vi "FOCUS_V42.vi"(9 "X-pixels":sgl=256.0, 11 "Run":bool) -> (0 "Retrace pixels":sgl, 10 "Pixel Clock (Hz)":sgl)   [LabVIEW 2010] (continued)
                  n1367 = property on="index (row)1" class="Slide (strict)"("Scale.Range:Minimum"=w940, "Scale.Range:Maximum"=w941) -> ()  [unwired: 2 in, 2 out]
                  n1368 = Add(x=w956, y=w957) -> (x+y=w955:dbl)
                  n1369 = property on="Histogram2" class="XYGraph (strict)"("X Scale.Range:Minimum"=w956, "X Scale.Range:Maximum"=w955) -> ()  [unwired: 2 in, 2 out]
                  n1370 = property on="Histogram1" class="XYGraph (strict)"("X Scale.Range:Minimum"=w956, "X Scale.Range:Maximum"=w955) -> ()  [unwired: 2 in, 2 out]
                  n1371 = Initialize Array(u32 0 ("element"), w891) -> (w949:u32[])
                  n1372 = Array Subset(array=w887, index (row)=w902, length (row)=w901) -> (w947:u8[][])  [unwired: 2 in]
                  n1373 = Initialize Array(u32 0 ("element"), w891) -> (w953:u32[])
                  n1374 = Array Subset(array=w886, index (row)=w900, length (row)=w899) -> (w951:u8[][])  [unwired: 2 in]
                  n1375 = property on="index (row)2" class="Slide (strict)"("Scale.Range:Minimum"=w940, "Scale.Range:Maximum"=w939) -> ()  [unwired: 2 in, 2 out]
                  n1376 = local read "Background1"() -> (w913:bool)
                  n1377 = for {
                    tunnel: w947 -> [w1024] mode=indexing
                    shift-right: [w1023] -> w948
                    shift-left: w949 -> [w1025]
                    n1378 = Add(x=w1025, y=w1024) -> (x+y=w1023:u32[])
                  }
                  n1379 = local read "Index1"() -> (w927:dbl)
                  n1380 = local read "Length1"() -> (w928:dbl)
                  n1381 = for {
                    tunnel: w951 -> [w1021] mode=indexing
                    shift-right: [w1020] -> w952
                    shift-left: w953 -> [w1022]
                    n1382 = Add(x=w1022, y=w1021) -> (x+y=w1020:u32[])
                  }
                  n1383 = local read "X-pixels"() -> (w889:sgl)
                  n1384 = local read "Pixel Clock (Hz)"() -> (w945:sgl)
                  n1385 = Divide(x=w948, y=w901) -> (x/y=w890:dbl[])
                  n1386 = Array Subset(array=w890, index=w927, length=w928) -> (w924:dbl[])
                  n1387 = Divide(x=w952, y=w899) -> (x/y=w930:dbl[])
                  n1388 = Array Subset(array=w887, index (row)=w956, length (row)=w957, index (col)=w903, length (col)=w888) -> (w959:u8[][])
                  n1389 = Array Subset(array=w886, index (row)=w956, length (row)=w957, index (col)=w903, length (col)=w888) -> (w958:u8[][])
                  n1390 = case shown="True" w913 {
                    tunnel: w890 -> [_ w967]
                    frame False {
                    }
                    frame True {
                      n1391 = Array Size(array=w967) -> (size(s)=w968:i32)
                      n1392 = Add Array Elements(numeric array=w967) -> (sum=w969:dbl)
                      n1393 = Divide(x=w969, y=w968) -> (x/y=w966:dbl)
                      n1394 = local write "Background1 2"(w966) -> ()
                    }
                  }
                  n1395 = Array Size(array=w924) -> (size(s)=w926:i32)
                  n1396 = Add Array Elements(numeric array=w924) -> (sum=w925:dbl)
                  n1397 = Divide(x=w889, y=w945) -> (x/y=w944:sgl)
                  n1398 = local write "Image 1"(w959) -> ()
                  n1399 = Divide(x=w925, y=w926) -> (x/y=w912:dbl)
                  n1400 = local write "Image 2"(w958) -> ()
                  n1401 = local write "F01 2"(w912) -> ()
                  n1402 = Multiply(x=1000.0, y=w944) -> (x*y=w894:dbl)
                  n1403 = Multiply(x=w891, y=w894) -> (x*y=w936:dbl)
                  n1404 = case shown="True" w914 {
                    tunnel: w936 -> [_ w1019]
                    frame False {
                    }
                    frame True {
                      n1405 = property on="Profile1" class="XYGraph (strict)"("X Scale.Range:Minimum"=0.0, "X Scale.Range:Maximum"=w1019, "Y Scale.Range:Minimum"=0.0, "Y Scale.Range:Maximum"=255.0) -> ()  [unwired: 2 in, 2 out]
                    }
                  }
                  n1406 = case shown="True" w915 {
                    tunnel: w936 -> [_ w996]
                    frame False {
                    }
                    frame True {
                      n1407 = property on="Profile2" class="XYGraph (strict)"("X Scale.Range:Minimum"=0.0, "X Scale.Range:Maximum"=w996, "Y Scale.Range:Minimum"=0.0, "Y Scale.Range:Maximum"=255.0) -> ()  [unwired: 2 in, 2 out]
                    }
                  }
                  n1408 = local read "F0 1"() -> (w907:bool)
                  n1409 = Multiply(x=w894, y=w942) -> (x*y=w896:dbl[])
                  n1410 = Multiply(x=w894, y=w942) -> (x*y=w954:dbl[])
                  n1411 = local read "F0 2"() -> (w908:bool)
                  n1412 = local read "Background2"() -> (w910:bool)
                  n1413 = case shown="True" w908 {
                    tunnel: w930 -> [w1000 w1014]
                    tunnel: [w1000 w1006] -> w938
                    tunnel: w904 -> [w999 _]
                    tunnel: [w997 i8 -1 ("Active Cursor")] -> w937
                    frame False {
                      n1414 = Less Than 0?(x=w999) -> (x < 0?=w998:bool)
                      n1415 = case shown="False" w998 {
                        selector: w998 -> [w1002 w1004]
                        tunnel: [i8 1 ("Active Cursor") i8 1 ("Active Cursor")] -> w997
                        frame False {
                          n1416 = local write "Reset2"(w1002) -> ()
                        }
                        frame True {
                          n1417 = local write "Reset2"(w1004) -> ()
                        }
                      }
                    }
                    frame True {
                      n1418 = local read "Background2 2"() -> (w1012:sgl)
                      n1419 = local read "F02 2"() -> (w1009:sgl)
                      n1420 = Subtract(x=w1014, y=w1009) -> (x-y=w1013:dbl[])
                      n1421 = Subtract(x=w1009, y=w1012) -> (x-y=w1015:sgl)
                      n1422 = Divide(x=w1013, y=w1015) -> (x/y=w1007:dbl[])
                      n1423 = property on="Profile2" class="XYGraph (strict)"("Y Scale.Range:Minimum"=-100.0, "Y Scale.Range:Maximum"=100.0) -> ()  [unwired: 2 in, 2 out]
                      n1424 = Multiply(x=w1007, y=100.0 ("Y Scale.Range:Maximum")) -> (x*y=w1006:dbl[])
                    }
                  }
                  n1425 = case shown="True" w907 {
                    tunnel: w890 -> [w973 w987]
                    tunnel: [w973 w979] -> w895
                    tunnel: w905 -> [w972 _]
                    tunnel: [w970 i8 -1 ("Active Cursor")] -> w929
                    frame False {
                      n1426 = Less Than 0?(x=w972) -> (x < 0?=w971:bool)
                      n1427 = case shown="True" w971 {
                        selector: w971 -> [w975 w977]
                        tunnel: [i8 1 ("Active Cursor") i8 1 ("Active Cursor")] -> w970
                        frame False {
                          n1428 = local write "Reset1"(w975) -> ()
                        }
                        frame True {
                          n1429 = local write "Reset1"(w977) -> ()
                        }
                      }
                    }
                    frame True {
                      n1430 = local read "Background1 2"() -> (w985:sgl)
                      n1431 = local read "F01 2"() -> (w982:sgl)
                      n1432 = Subtract(x=w987, y=w982) -> (x-y=w986:dbl[])
                      n1433 = Subtract(x=w982, y=w985) -> (x-y=w988:sgl)
                      n1434 = Divide(x=w986, y=w988) -> (x/y=w980:dbl[])
                      n1435 = property on="Profile1" class="XYGraph (strict)"("Y Scale.Range:Minimum"=-100.0, "Y Scale.Range:Maximum"=100.0) -> ()  [unwired: 2 in, 2 out]
                      n1436 = Multiply(x=w980, y=100.0 ("Y Scale.Range:Maximum")) -> (x*y=w979:dbl[])
                    }
                  }
                  n1437 = property on="Profile2" class="XYGraph (strict)"() -> ("X Scale.Range:Minimum"=w919:dbl, "X Scale.Range:Maximum"=w918:dbl)  [unwired: 2 in, 2 out]
                  n1438 = local read "Index2"() -> (w932:dbl)
                  n1439 = local read "Length2"() -> (w931:dbl)
                  n1440 = property on="Profile1" class="XYGraph (strict)"() -> ("X Scale.Range:Minimum"=w920:dbl, "X Scale.Range:Maximum"=w921:dbl)  [unwired: 2 in, 2 out]
                  n1441 = case shown="True" w910 {
                    tunnel: w930 -> [_ w990]
                    frame False {
                    }
                    frame True {
                      n1442 = Array Size(array=w990) -> (size(s)=w991:i32)
                      n1443 = Add Array Elements(numeric array=w990) -> (sum=w992:dbl)
                      n1444 = Divide(x=w992, y=w991) -> (x/y=w989:dbl)
                      n1445 = local write "Background2 2"(w989) -> ()
                    }
                  }
                  n1446 = Array Subset(array=w930, index=w932, length=w931) -> (w935:dbl[])
                  n1447 = local read "F02"() -> (w906:bool)
                  n1448 = local read "F01"() -> (w911:bool)
                  n1449 = Divide(x=w919, y=w894) -> (x/y=w917:dbl)
                  n1450 = Divide(x=w918, y=w894) -> (x/y=w916:dbl)
                  n1451 = Divide(x=w920, y=w894) -> (x/y=w922:dbl)
                  n1452 = Divide(x=w921, y=w894) -> (x/y=w923:dbl)
                  n1453 = Array Size(array=w935) -> (size(s)=w933:i32)
                  n1454 = Add Array Elements(numeric array=w935) -> (sum=w934:dbl)
                  n1455 = case shown="True" w906 {
                    tunnel: w917 -> [_ w961]
                    tunnel: w916 -> [_ w962]
                    frame False {
                    }
                    frame True {
                      n1456 = local write "Index2"(w961) -> ()
                      n1457 = Subtract(x=w962, y=w961) -> (x-y=w960:dbl)
                      n1458 = local write "Length2"(w960) -> ()
                    }
                  }
                  n1459 = case shown="True" w911 {
                    tunnel: w922 -> [_ w964]
                    tunnel: w923 -> [_ w965]
                    frame False {
                    }
                    frame True {
                      n1460 = Subtract(x=w965, y=w964) -> (x-y=w963:dbl)
                      n1461 = local write "Index1"(w964) -> ()
                      n1462 = local write "Length1"(w963) -> ()
                    }
                  }
                  n1463 = Divide(x=w934, y=w933) -> (x/y=w909:dbl)
                  n1464 = local write "F02 2"(w909) -> ()
                  n1465 = Bundle(w954, w938) -> (w898:cluster{dbl[], dbl[]})  [unwired: 1 in]
                  n1466 = local write "Profile2"(w898) -> ()
                  n1467 = Bundle(w896, w895) -> (w897:cluster{dbl[], dbl[]})  [unwired: 1 in]
                  n1468 = local write "Profile1"(w897) -> ()
                }
                frame True {
                  n1469 = local read "Y-Scale"() -> (w1028:bool)
                  n1470 = case shown="False" w1028 {
                    tunnel: w1027 -> [w1030 _]
                    tunnel: w1026 -> [w1029 _]
                    frame False {
                      n1471 = local read "Y-lines"() -> (w1032:sgl)
                      n1472 = local read "Number of frames"() -> (w1033:sgl)
                      n1473 = local read "X-pixels"() -> (w1035:sgl)
                      n1474 = Multiply(x=w1033, y=w1032) -> (x*y=w1031:sgl)
                      n1475 = Subtract(x=w1031, y=w1035) -> (x-y=w1034:sgl)
                      n1476 = while {
                        shift-right: [w1044] -> _
                        shift-left: i16 0 ("y") -> [w1045]
                        tunnel: w1034 -> [w1043]
                        tunnel: w1030 -> [w1038]
                        tunnel: w1029 -> [w1037]
                        stop <- w1041 stop-if-true
                        n1477 = call "ResetToZeroFOCUS.vi"("UpperLimit"=w1043, "Running Index"=w1045) -> ("New Index"=w1039:i32)
                        n1478 = local read "Play Movie"() -> (w1042:bool)
                        n1479 = local write "ImageSlide"(w1039) -> ()
                        n1480 = local read "X-pixels"() -> (w1048:sgl)
                        n1481 = Not(x=w1042) -> (.not. x?=w1041:bool)
                        n1482 = Increment(x=w1039) -> (x+1=w1044:i32)
                        n1483 = local read "Velocity"() -> (w1040:dbl)
                        n1484 = Array Subset(array=w1038, index (col)=w1039, length (col)=w1048) -> (w1047:u8[][])  [unwired: 2 in]
                        n1485 = Array Subset(array=w1037, index (col)=w1039, length (col)=w1048) -> (w1046:u8[][])  [unwired: 2 in]
                        n1486 = Wait Until Next ms Multiple(millisecond multiple=w1040) -> ()  [unwired: 1 out]
                        n1487 = local write "Image 1"(w1047) -> ()
                        n1488 = local write "Image 2"(w1046) -> ()
                      }
                    }
                    frame True {
                    }
                  }
                }
              }
            }
            frame 3 {
              n1489 = case shown="False" w1055 {
                tunnel: w1054 -> [_ _]
                tunnel: w1060 -> [w1119 _]
                tunnel: [w1113 _] -> w1057
                tunnel: [w1105 _] -> w1056
                tunnel: w1059 -> [w1074 _]
                tunnel: w1058 -> [w1073 _]
                tunnel: w1053 -> [w1065 _]
                tunnel: w1052 -> [w1064 w1205]
                tunnel: w1051 -> [w1063 w1204]
                tunnel: w1050 -> [w1062 _]
                tunnel: w1049 -> [w1061 _]
                frame False {
                  w1066 = 0 ("index")
                  w1134 = 0.0
                  w1117 = 0.0 ("Scale.Range:Minimum")
                  n1490 = local read "Reset1"() -> (w1089:bool)
                  n1491 = local read "Reset2"() -> (w1090:bool)
                  n1492 = local read "Y-lines FreeLine"() -> (w1115:sgl)
                  n1493 = local read "X-pixels FreeLine"() -> (w1135:sgl)
                  n1494 = Add(x=w1134, y=w1135) -> (x+y=w1133:dbl)
                  n1495 = property on="Histogram2" class="XYGraph (strict)"("X Scale.Range:Minimum"=w1134, "X Scale.Range:Maximum"=w1133) -> ()  [unwired: 2 in, 2 out]
                  n1496 = property on="Histogram1" class="XYGraph (strict)"("X Scale.Range:Minimum"=w1134, "X Scale.Range:Maximum"=w1133) -> ()  [unwired: 2 in, 2 out]
                  n1497 = Initialize Array(u32 0 ("element"), w1115) -> (w1127:u32[])
                  n1498 = Array Subset(array=w1064, index (row)="index (row)1", length (row)="Average1") -> (w1125:u8[][])  [unwired: 2 in]
                  n1499 = Initialize Array(u32 0 ("element"), w1115) -> (w1131:u32[])
                  n1500 = Array Subset(array=w1063, index (row)="index (row)2", length (row)="Average2") -> (w1129:u8[][])  [unwired: 2 in]
                  n1501 = local read "Background1"() -> (w1088:bool)
                  n1502 = for {
                    tunnel: w1125 -> [w1202] mode=indexing
                    shift-right: [w1201] -> w1126
                    shift-left: w1127 -> [w1203]
                    n1503 = Add(x=w1203, y=w1202) -> (x+y=w1201:u32[])
                  }
                  n1504 = local read "Index1"() -> (w1103:dbl)
                  n1505 = local read "Length1"() -> (w1104:dbl)
                  n1506 = for {
                    tunnel: w1129 -> [w1199] mode=indexing
                    shift-right: [w1198] -> w1130
                    shift-left: w1131 -> [w1200]
                    n1507 = Add(x=w1200, y=w1199) -> (x+y=w1198:u32[])
                  }
                  n1508 = local read "X-pixels FreeLine"() -> (w1067:sgl)
                  n1509 = Subtract(x=w1067, y="Average2") -> (x-y=w1116:sgl)
                  n1510 = Subtract(x=w1067, y="Average1") -> (x-y=w1118:sgl)
                  n1511 = property on="index (row)1" class="Slide (strict)"("Scale.Range:Minimum"=w1117, "Scale.Range:Maximum"=w1118) -> ()  [unwired: 2 in, 2 out]
                  n1512 = property on="index (row)2" class="Slide (strict)"("Scale.Range:Minimum"=w1117, "Scale.Range:Maximum"=w1116) -> ()  [unwired: 2 in, 2 out]
                  n1513 = local read "Pixel Clock (Hz) FreeLine"() -> (w1123:sgl)
                  n1514 = Divide(x=w1126, y="Average1") -> (x/y=w1072:dbl[])
                  n1515 = Array Subset(array=w1072, index=w1103, length=w1104) -> (w1100:dbl[])
                  n1516 = Divide(x=w1130, y="Average2") -> (x/y=w1106:dbl[])
                  n1517 = Array Subset(array=w1064, index (row)=w1134, length (row)=w1135, index (col)=w1065, length (col)=w1067) -> (w1137:u8[][])
                  n1518 = Array Subset(array=w1063, index (row)=w1134, length (row)=w1135, index (col)=w1065, length (col)=w1067) -> (w1136:u8[][])
                  n1519 = case shown="True" w1088 {
                    tunnel: w1072 -> [_ w1145]
                    frame False {
                    }
                    frame True {
                      n1520 = Array Size(array=w1145) -> (size(s)=w1146:i32)
                      n1521 = Add Array Elements(numeric array=w1145) -> (sum=w1147:dbl)
                      n1522 = Divide(x=w1147, y=w1146) -> (x/y=w1144:dbl)
                      n1523 = local write "Background1 2"(w1144) -> ()
                    }
                  }
                  n1524 = Array Size(array=w1100) -> (size(s)=w1102:i32)
                  n1525 = Add Array Elements(numeric array=w1100) -> (sum=w1101:dbl)
                  n1526 = Divide(x=w1067, y=w1123) -> (x/y=w1122:sgl)
                  n1527 = local write "Image 3"(w1137) -> ()
                  n1528 = Divide(x=w1101, y=w1102) -> (x/y=w1087:dbl)
                  n1529 = local write "Image 4"(w1136) -> ()
                  n1530 = local write "F01 2"(w1087) -> ()
                  n1531 = Multiply(x=1000.0, y=w1122) -> (x*y=w1091:dbl)
                  n1532 = Multiply(x=w1115, y=w1091) -> (x*y=w1112:dbl)
                  n1533 = case shown="True" w1089 {
                    tunnel: w1112 -> [_ w1197]
                    frame False {
                    }
                    frame True {
                      n1534 = property on="Profile1" class="XYGraph (strict)"("X Scale.Range:Minimum"=0.0, "X Scale.Range:Maximum"=w1197, "Y Scale.Range:Minimum"=0.0, "Y Scale.Range:Maximum"=255.0) -> ()  [unwired: 2 in, 2 out]
                    }
                  }
                  n1535 = case shown="True" w1090 {
                    tunnel: w1112 -> [_ w1174]
                    frame False {
                    }
                    frame True {
                      n1536 = property on="Profile2" class="XYGraph (strict)"("X Scale.Range:Minimum"=0.0, "X Scale.Range:Maximum"=w1174, "Y Scale.Range:Minimum"=0.0, "Y Scale.Range:Maximum"=255.0) -> ()  [unwired: 2 in, 2 out]
                    }
                  }
                  n1537 = local read "Y-lines"() -> (w1068:sgl)
                  n1538 = local read "F0 1"() -> (w1082:bool)
                  n1539 = Multiply(x=w1091, y=w1119) -> (x*y=w1120:dbl[])
                  n1540 = Multiply(x=w1091, y=w1119) -> (x*y=w1132:dbl[])
                  n1541 = local read "F0 2"() -> (w1083:bool)
                  n1542 = local read "Background2"() -> (w1085:bool)
                  n1543 = case shown="True" w1083 {
                    tunnel: w1106 -> [w1178 w1192]
                    tunnel: [w1178 w1184] -> w1114
                    tunnel: w1073 -> [w1177 _]
                    tunnel: [w1175 i8 -1 ("Active Cursor")] -> w1113
                    frame False {
                      n1544 = Less Than 0?(x=w1177) -> (x < 0?=w1176:bool)
                      n1545 = case shown="True" w1176 {
                        selector: w1176 -> [w1180 w1182]
                        tunnel: [i8 1 ("Active Cursor") i8 1 ("Active Cursor")] -> w1175
                        frame False {
                          n1546 = local write "Reset2"(w1180) -> ()
                        }
                        frame True {
                          n1547 = local write "Reset2"(w1182) -> ()
                        }
                      }
                    }
                    frame True {
                      n1548 = local read "Background2 2"() -> (w1190:sgl)
                      n1549 = local read "F02 2"() -> (w1187:sgl)
                      n1550 = Subtract(x=w1192, y=w1187) -> (x-y=w1191:dbl[])
                      n1551 = Subtract(x=w1187, y=w1190) -> (x-y=w1193:sgl)
                      n1552 = Divide(x=w1191, y=w1193) -> (x/y=w1185:dbl[])
                      n1553 = property on="Profile2" class="XYGraph (strict)"("Y Scale.Range:Minimum"=-100.0, "Y Scale.Range:Maximum"=100.0) -> ()  [unwired: 2 in, 2 out]
                      n1554 = Multiply(x=w1185, y=100.0 ("Y Scale.Range:Maximum")) -> (x*y=w1184:dbl[])
                    }
                  }
                  n1555 = case shown="True" w1082 {
                    tunnel: w1072 -> [w1151 w1165]
                    tunnel: [w1151 w1157] -> w1071
                    tunnel: w1074 -> [w1150 _]
                    tunnel: [w1148 i8 -1 ("Active Cursor")] -> w1105
                    frame False {
                      n1556 = Less Than 0?(x=w1150) -> (x < 0?=w1149:bool)
                      n1557 = case shown="False" w1149 {
                        selector: w1149 -> [w1153 w1155]
                        tunnel: [i8 1 ("Active Cursor") i8 1 ("Active Cursor")] -> w1148
                        frame False {
                          n1558 = local write "Reset1"(w1153) -> ()
                        }
                        frame True {
                          n1559 = local write "Reset1"(w1155) -> ()
                        }
                      }
                    }
                    frame True {
                      n1560 = local read "Background1 2"() -> (w1163:sgl)
                      n1561 = local read "F01 2"() -> (w1160:sgl)
                      n1562 = Subtract(x=w1165, y=w1160) -> (x-y=w1164:dbl[])
                      n1563 = Subtract(x=w1160, y=w1163) -> (x-y=w1166:sgl)
                      n1564 = Divide(x=w1164, y=w1166) -> (x/y=w1158:dbl[])
                      n1565 = property on="Profile1" class="XYGraph (strict)"("Y Scale.Range:Minimum"=-100.0, "Y Scale.Range:Maximum"=100.0) -> ()  [unwired: 2 in, 2 out]
                      n1566 = Multiply(x=w1158, y=100.0 ("Y Scale.Range:Maximum")) -> (x*y=w1157:dbl[])
                    }
                  }
                  n1567 = property on="Profile2" class="XYGraph (strict)"() -> ("X Scale.Range:Minimum"=w1095:dbl, "X Scale.Range:Maximum"=w1094:dbl)  [unwired: 2 in, 2 out]
                  n1568 = Array Subset(array=w1062, index (col)=w1066, length (col)=w1068) -> (w1070:u8[][])  [unwired: 2 in]
                  n1569 = local read "Index2"() -> (w1108:dbl)
                  n1570 = local read "Length2"() -> (w1107:dbl)
                  n1571 = property on="Profile1" class="XYGraph (strict)"() -> ("X Scale.Range:Minimum"=w1096:dbl, "X Scale.Range:Maximum"=w1097:dbl)  [unwired: 2 in, 2 out]
                  n1572 = local write "Image 1"(w1070) -> ()
                  n1573 = case shown="True" w1085 {
                    tunnel: w1106 -> [_ w1168]
                    frame False {
                    }
                    frame True {
                      n1574 = Array Size(array=w1168) -> (size(s)=w1169:i32)
                      n1575 = Add Array Elements(numeric array=w1168) -> (sum=w1170:dbl)
                      n1576 = Divide(x=w1170, y=w1169) -> (x/y=w1167:dbl)
                      n1577 = local write "Background2 2"(w1167) -> ()
                    }
                  }
                  n1578 = Array Subset(array=w1106, index=w1108, length=w1107) -> (w1111:dbl[])
                  n1579 = local read "F02"() -> (w1081:bool)
                  n1580 = local read "F01"() -> (w1086:bool)
                  n1581 = Divide(x=w1095, y=w1091) -> (x/y=w1093:dbl)
                  n1582 = Divide(x=w1094, y=w1091) -> (x/y=w1092:dbl)
                  n1583 = Divide(x=w1096, y=w1091) -> (x/y=w1098:dbl)
                  n1584 = Divide(x=w1097, y=w1091) -> (x/y=w1099:dbl)
                  n1585 = Array Size(array=w1111) -> (size(s)=w1109:i32)
                  n1586 = Add Array Elements(numeric array=w1111) -> (sum=w1110:dbl)
                  n1587 = case shown="True" w1081 {
                    tunnel: w1093 -> [_ w1139]
                    tunnel: w1092 -> [_ w1140]
                    frame False {
                    }
                    frame True {
                      n1588 = local write "Index2"(w1139) -> ()
                      n1589 = Subtract(x=w1140, y=w1139) -> (x-y=w1138:dbl)
                      n1590 = local write "Length2"(w1138) -> ()
                    }
                  }
                  n1591 = case shown="True" w1086 {
                    tunnel: w1098 -> [_ w1142]
                    tunnel: w1099 -> [_ w1143]
                    frame False {
                    }
                    frame True {
                      n1592 = Subtract(x=w1143, y=w1142) -> (x-y=w1141:dbl)
                      n1593 = local write "Index1"(w1142) -> ()
                      n1594 = local write "Length1"(w1141) -> ()
                    }
                  }
                  n1595 = Divide(x=w1110, y=w1109) -> (x/y=w1084:dbl)
                  n1596 = Array Subset(array=w1061, index (col)=w1066, length (col)=w1068) -> (w1069:u8[][])  [unwired: 2 in]
                  n1597 = local write "F02 2"(w1084) -> ()
                  n1598 = local write "Image 2"(w1069) -> ()
                  n1599 = Bundle(w1132, w1114) -> (→"Profile2":cluster{dbl[], dbl[]})  [unwired: 1 in]
                  n1600 = Bundle(w1120, w1071) -> (→"Profile1":cluster{dbl[], dbl[]})  [unwired: 1 in]
                }
                frame True {
                  n1601 = local read "X-pixels FreeLine"() -> (w1208:sgl)
                  n1602 = local read "Y-lines FreeLine"() -> (w1206:sgl)
                  n1603 = Subtract(x=w1206, y=w1208) -> (x-y=w1207:sgl)
                  n1604 = while {
                    shift-right: [w1218] -> _
                    shift-left: i16 0 ("y") -> [w1219]
                    tunnel: w1207 -> [w1217]
                    tunnel: w1206 -> [w1213]
                    tunnel: w1205 -> [w1211]
                    tunnel: w1204 -> [w1210]
                    stop <- w1215 stop-if-true
                    n1605 = call "ResetToZeroFOCUS.vi"("UpperLimit"=w1217, "Running Index"=w1219) -> ("New Index"=w1212:i32)
                    n1606 = Multiply(x=w1212, y=w1213) -> ()  [unwired: 1 out]
                    n1607 = local read "Play Movie"() -> (w1216:bool)
                    n1608 = local write "ImageSlide"(w1212) -> ()
                    n1609 = local read "X-pixels FreeLine"() -> (w1222:sgl)
                    n1610 = Not(x=w1216) -> (.not. x?=w1215:bool)
                    n1611 = Increment(x=w1212) -> (x+1=w1218:i32)
                    n1612 = local read "Velocity"() -> (w1214:dbl)
                    n1613 = Array Subset(array=w1211, index (col)=w1212, length (col)=w1222) -> (w1221:u8[][])  [unwired: 2 in]
                    n1614 = Array Subset(array=w1210, index (col)=w1212, length (col)=w1222) -> (w1220:u8[][])  [unwired: 2 in]
                    n1615 = Wait Until Next ms Multiple(millisecond multiple=w1214) -> ()  [unwired: 1 out]
                    n1616 = local write "Image 3"(w1221) -> ()
                    n1617 = local write "Image 4"(w1220) -> ()
                  }
                }
              }
            }
            frame 4 {
              n1618 = case shown="False" w1233 {
                tunnel: w1234 -> [w1239 _]
                tunnel: w1232 -> [w1314 _]
                tunnel: w1231 -> [w1294 _]
                tunnel: w1230 -> [w1280 _]
                tunnel: [w1279 _] -> w1229
                tunnel: w1228 -> [w1268 _]
                tunnel: [w1267 _] -> w1227
                tunnel: w1226 -> [w1238 w1388]
                tunnel: w1225 -> [w1237 w1387]
                tunnel: w1224 -> [w1236 _]
                tunnel: w1223 -> [w1235 _]
                frame False {
                  w1291 = 0.0 ("Scale.Range:Minimum")
                  n1619 = local read "index (row)2"() -> (w1289:i32)
                  n1620 = local read "XScale"() -> (w1313:bool)
                  n1621 = local read "index (row)1"() -> (w1287:i32)
                  n1622 = Round To Nearest(number=w1314) -> (nearest integer value=w1312:u32)
                  n1623 = local read "Y-lines FreeLine"() -> (w1283:sgl)
                  n1624 = case shown="False" w1313 {
                    tunnel: [w1384 w1386] -> w1311
                    tunnel: w1312 -> [w1383 _]
                    tunnel: [w1383 0.0] -> w1310
                    frame False {
                      n1625 = local read "Y-lines FreeLine"() -> (w1384:sgl)
                    }
                    frame True {
                      n1626 = local read "X-pixels FreeLine"() -> (w1386:sgl)
                    }
                  }
                  n1627 = local read "Average2"() -> (w1286:i32)
                  n1628 = local read "Average1"() -> (w1285:i32)
                  n1629 = Add(x=w1310, y=w1311) -> (x+y=w1309:dbl)
                  n1630 = property on="Histogram2" class="XYGraph (strict)"("X Scale.Range:Minimum"=w1310, "X Scale.Range:Maximum"=w1309) -> ()  [unwired: 2 in, 2 out]
                  n1631 = property on="Histogram1" class="XYGraph (strict)"("X Scale.Range:Minimum"=w1310, "X Scale.Range:Maximum"=w1309) -> ()  [unwired: 2 in, 2 out]
                  n1632 = Initialize Array(u32 0 ("element"), w1283) -> (w1303:u32[])
                  n1633 = Array Subset(array=w1238, index (row)=w1287, length (row)=w1285) -> (w1301:u8[][])  [unwired: 2 in]
                  n1634 = Initialize Array(u32 0 ("element"), w1283) -> (w1307:u32[])
                  n1635 = Array Subset(array=w1237, index (row)=w1289, length (row)=w1286) -> (w1305:u8[][])  [unwired: 2 in]
                  n1636 = for {
                    tunnel: w1301 -> [w1381] mode=indexing
                    shift-right: [w1380] -> w1302
                    shift-left: w1303 -> [w1382]
                    n1637 = Add(x=w1382, y=w1381) -> (x+y=w1380:u32[])
                  }
                  n1638 = local read "Index1"() -> (w1263:dbl)
                  n1639 = local read "Length1"() -> (w1264:dbl)
                  n1640 = for {
                    tunnel: w1305 -> [w1378] mode=indexing
                    shift-right: [w1377] -> w1306
                    shift-left: w1307 -> [w1379]
                    n1641 = Add(x=w1379, y=w1378) -> (x+y=w1377:u32[])
                  }
                  n1642 = local read "X-pixels FreeLine"() -> (w1290:sgl)
                  n1643 = Subtract(x=w1290, y=w1286) -> (x-y=w1288:sgl)
                  n1644 = Subtract(x=w1290, y=w1285) -> (x-y=w1292:sgl)
                  n1645 = property on="index (row)1" class="Slide (strict)"("Scale.Range:Minimum"=w1291, "Scale.Range:Maximum"=w1292) -> ()  [unwired: 2 in, 2 out]
                  n1646 = property on="index (row)2" class="Slide (strict)"("Scale.Range:Minimum"=w1291, "Scale.Range:Maximum"=w1288) -> ()  [unwired: 2 in, 2 out]
                  n1647 = local read "Pixel Clock (Hz) FreeLine"() -> (w1299:sgl)
                  n1648 = Divide(x=w1302, y=w1285) -> (x/y=w1247:dbl[])
                  n1649 = Array Subset(array=w1247, index=w1263, length=w1264) -> (w1259:dbl[])
                  n1650 = Divide(x=w1306, y=w1286) -> (x/y=w1269:dbl[])
                  n1651 = Array Subset(array=w1238, index (row)=w1310, length (row)=w1311) -> (w1316:u8[][])  [unwired: 2 in]
                  n1652 = Array Subset(array=w1237, index (row)=w1310, length (row)=w1311) -> (w1315:u8[][])  [unwired: 2 in]
                  n1653 = local read "Y-lines"() -> (w1245:sgl)
                  n1654 = case shown="True" "Background1" {
                    tunnel: w1247 -> [_ w1324]
                    frame False {
                    }
                    frame True {
                      n1655 = Array Size(array=w1324) -> (size(s)=w1325:i32)
                      n1656 = Add Array Elements(numeric array=w1324) -> (sum=w1326:dbl)
                      n1657 = Divide(x=w1326, y=w1325) -> (x/y=→"Background1 2":dbl)
                    }
                  }
                  n1658 = Array Size(array=w1259) -> (size(s)=w1262:i32)
                  n1659 = Add Array Elements(numeric array=w1259) -> (sum=w1261:dbl)
                  n1660 = Round To Nearest(number=w1239) -> (nearest integer value=w1244:u32)
                  n1661 = Divide(x=w1290, y=w1299) -> (x/y=w1298:sgl)
                  n1662 = local write "Image 3"(w1316) -> ()
                  n1663 = Divide(x=w1261, y=w1262) -> (x/y=→"F01 2":dbl)
                  n1664 = local write "Image 4"(w1315) -> ()
                  n1665 = Multiply(x=w1245, y=w1244) -> (x*y=w1240:sgl)
                  n1666 = local read "Y-lines"() -> (w1241:sgl)
                  n1667 = Multiply(x=1000.0, y=w1298) -> (x*y=w1248:dbl)
                  n1668 = Multiply(x=w1283, y=w1248) -> (x*y=w1278:dbl)
                  n1669 = case shown="True" "Reset1" {
                    tunnel: w1278 -> [_ w1376]
                    frame False {
                    }
                    frame True {
                      n1670 = property on="Profile1" class="XYGraph (strict)"("X Scale.Range:Minimum"=0.0, "X Scale.Range:Maximum"=w1376, "Y Scale.Range:Minimum"=0.0, "Y Scale.Range:Maximum"=255.0) -> ()  [unwired: 2 in, 2 out]
                    }
                  }
                  n1671 = case shown="True" "Reset2" {
                    tunnel: w1278 -> [_ w1353]
                    frame False {
                    }
                    frame True {
                      n1672 = property on="Profile2" class="XYGraph (strict)"("X Scale.Range:Minimum"=0.0, "X Scale.Range:Maximum"=w1353, "Y Scale.Range:Minimum"=0.0, "Y Scale.Range:Maximum"=255.0) -> ()  [unwired: 2 in, 2 out]
                    }
                  }
                  n1673 = Multiply(x=w1248, y=w1294) -> (x*y=w1295:dbl[])
                  n1674 = Multiply(x=w1248, y=w1294) -> (x*y=w1308:dbl[])
                  n1675 = Array Subset(array=w1236, index (col)=w1240, length (col)=w1241) -> (w1243:u8[][])  [unwired: 2 in]
                  n1676 = case shown="True" "F0 1" {
                    tunnel: w1247 -> [w1330 w1344]
                    tunnel: [w1330 w1336] -> w1246
                    tunnel: w1268 -> [w1329 _]
                    tunnel: [w1327 i8 -1 ("Active Cursor")] -> w1267
                    frame False {
                      n1677 = Less Than 0?(x=w1329) -> (x < 0?=w1328:bool)
                      n1678 = case shown="True" w1328 {
                        selector: w1328 -> [w1332 w1334]
                        tunnel: [i8 1 ("Active Cursor") i8 1 ("Active Cursor")] -> w1327
                        frame False {
                          n1679 = local write "Reset1"(w1332) -> ()
                        }
                        frame True {
                          n1680 = local write "Reset1"(w1334) -> ()
                        }
                      }
                    }
                    frame True {
                      n1681 = local read "Background1 2"() -> (w1342:sgl)
                      n1682 = local read "F01 2"() -> (w1339:sgl)
                      n1683 = Subtract(x=w1344, y=w1339) -> (x-y=w1343:dbl[])
                      n1684 = Subtract(x=w1339, y=w1342) -> (x-y=w1345:sgl)
                      n1685 = Divide(x=w1343, y=w1345) -> (x/y=w1337:dbl[])
                      n1686 = property on="Profile1" class="XYGraph (strict)"("Y Scale.Range:Minimum"=-100.0, "Y Scale.Range:Maximum"=100.0) -> ()  [unwired: 2 in, 2 out]
                      n1687 = Multiply(x=w1337, y=100.0 ("Y Scale.Range:Maximum")) -> (x*y=w1336:dbl[])
                    }
                  }
                  n1688 = case shown="True" "F0 2" {
                    tunnel: w1269 -> [w1357 w1371]
                    tunnel: [w1357 w1363] -> w1281
                    tunnel: w1280 -> [w1356 _]
                    tunnel: [w1354 i8 -1 ("Active Cursor")] -> w1279
                    frame False {
                      n1689 = Less Than 0?(x=w1356) -> (x < 0?=w1355:bool)
                      n1690 = case shown="False" w1355 {
                        selector: w1355 -> [w1359 w1361]
                        tunnel: [i8 1 ("Active Cursor") i8 1 ("Active Cursor")] -> w1354
                        frame False {
                          n1691 = local write "Reset2"(w1359) -> ()
                        }
                        frame True {
                          n1692 = local write "Reset2"(w1361) -> ()
                        }
                      }
                    }
                    frame True {
                      n1693 = local read "Background2 2"() -> (w1369:sgl)
                      n1694 = local read "F02 2"() -> (w1366:sgl)
                      n1695 = Subtract(x=w1371, y=w1366) -> (x-y=w1370:dbl[])
                      n1696 = Subtract(x=w1366, y=w1369) -> (x-y=w1372:sgl)
                      n1697 = Divide(x=w1370, y=w1372) -> (x/y=w1364:dbl[])
                      n1698 = property on="Profile2" class="XYGraph (strict)"("Y Scale.Range:Minimum"=-100.0, "Y Scale.Range:Maximum"=100.0) -> ()  [unwired: 2 in, 2 out]
                      n1699 = Multiply(x=w1364, y=100.0 ("Y Scale.Range:Maximum")) -> (x*y=w1363:dbl[])
                    }
                  }
                  n1700 = local read "Index2"() -> (w1272:dbl)
                  n1701 = local read "Length2"() -> (w1271:dbl)
                  n1702 = property on="Profile1" class="XYGraph (strict)"() -> ("X Scale.Range:Minimum"=w1254:dbl, "X Scale.Range:Maximum"=w1255:dbl)  [unwired: 2 in, 2 out]
                  n1703 = local write "Image 1"(w1243) -> ()
                  n1704 = property on="Profile2" class="XYGraph (strict)"() -> ("X Scale.Range:Minimum"=w1253:dbl, "X Scale.Range:Maximum"=w1252:dbl)  [unwired: 2 in, 2 out]
                  n1705 = case shown="True" "Background2" {
                    tunnel: w1269 -> [_ w1347]
                    frame False {
                    }
                    frame True {
                      n1706 = Array Size(array=w1347) -> (size(s)=w1348:i32)
                      n1707 = Add Array Elements(numeric array=w1347) -> (sum=w1349:dbl)
                      n1708 = Divide(x=w1349, y=w1348) -> (x/y=→"Background2 2":dbl)
                    }
                  }
                  n1709 = Array Subset(array=w1269, index=w1272, length=w1271) -> (w1276:dbl[])
                  n1710 = Divide(x=w1254, y=w1248) -> (x/y=w1257:dbl)
                  n1711 = Divide(x=w1255, y=w1248) -> (x/y=w1258:dbl)
                  n1712 = Array Size(array=w1276) -> (size(s)=w1273:i32)
                  n1713 = Add Array Elements(numeric array=w1276) -> (sum=w1274:dbl)
                  n1714 = Divide(x=w1253, y=w1248) -> (x/y=w1250:dbl)
                  n1715 = Divide(x=w1252, y=w1248) -> (x/y=w1249:dbl)
                  n1716 = case shown="True" "F01" {
                    tunnel: w1257 -> [_ w1321]
                    tunnel: w1258 -> [_ w1322]
                    frame False {
                    }
                    frame True {
                      n1717 = Subtract(x=w1322, y=w1321) -> (x-y=→"Length1":dbl)
                      "Index1" <- w1321
                    }
                  }
                  n1718 = Divide(x=w1274, y=w1273) -> (x/y=→"F02 2":dbl)
                  n1719 = Array Subset(array=w1235, index (col)=w1240, length (col)=w1241) -> (w1242:u8[][])  [unwired: 2 in]
                  n1720 = case shown="True" "F02" {
                    tunnel: w1250 -> [_ w1318]
                    tunnel: w1249 -> [_ w1319]
                    frame False {
                    }
                    frame True {
                      n1721 = Subtract(x=w1319, y=w1318) -> (x-y=→"Length2":dbl)
                      "Index2" <- w1318
                    }
                  }
                  n1722 = local write "Image 2"(w1242) -> ()
                  n1723 = Bundle(w1308, w1281) -> (w1296:cluster{dbl[], dbl[]})  [unwired: 1 in]
                  n1724 = local write "Profile2"(w1296) -> ()
                  n1725 = Bundle(w1295, w1246) -> (w1293:cluster{dbl[], dbl[]})  [unwired: 1 in]
                  n1726 = local write "Profile1"(w1293) -> ()
                }
                frame True {
                  n1727 = local read "X-pixels FreeLine"() -> (w1391:sgl)
                  n1728 = local read "Y-lines FreeLine"() -> (w1389:sgl)
                  n1729 = Subtract(x=w1389, y=w1391) -> (x-y=w1390:sgl)
                  n1730 = while {
                    shift-right: [w1401] -> _
                    shift-left: i16 0 ("y") -> [w1402]
                    tunnel: w1390 -> [w1400]
                    tunnel: w1389 -> [w1396]
                    tunnel: w1388 -> [w1394]
                    tunnel: w1387 -> [w1393]
                    stop <- w1398 stop-if-true
                    n1731 = call "ResetToZeroFOCUS.vi"("UpperLimit"=w1400, "Running Index"=w1402) -> ("New Index"=w1395:i32)
                    n1732 = Multiply(x=w1395, y=w1396) -> ()  [unwired: 1 out]
                    n1733 = local read "Play Movie"() -> (w1399:bool)
                    n1734 = local write "ImageSlide"(w1395) -> ()
                    n1735 = local read "Y-lines FreeLine"() -> (w1405:sgl)
                    n1736 = Not(x=w1399) -> (.not. x?=w1398:bool)
                    n1737 = Increment(x=w1395) -> (x+1=w1401:i32)
                    n1738 = local read "Velocity"() -> (w1397:dbl)
                    n1739 = Array Subset(array=w1394, index (col)=w1395, length (col)=w1405) -> (w1404:u8[][])  [unwired: 2 in]
                    n1740 = Array Subset(array=w1393, index (col)=w1395, length (col)=w1405) -> (w1403:u8[][])  [unwired: 2 in]
                    n1741 = Wait Until Next ms Multiple(millisecond multiple=w1397) -> ()  [unwired: 1 out]
                    n1742 = local write "Image 3"(w1404) -> ()
                    n1743 = local write "Image 4"(w1403) -> ()
                  }
                }
              }
            }
          }
          n1744 = property on="Image 2" class="IntGraph (strict)"("Y Scale.Range:Maximum"=w499) -> ()  [unwired: 2 in, 2 out]
          n1745 = property on="SlideHorizontal" class="Slide (strict)"("Visible"=w569) -> ()  [unwired: 2 in, 2 out]
          n1746 = case shown="True" w519 {
            tunnel: w530 -> [_ w817]
            tunnel: "ImageSelector" -> [_ w815]
            tunnel: [w814 w815] -> w528
            tunnel: w527 -> [w814 _]
            frame False {
            }
            frame True {
              n1747 = Round Toward +Infinity(x=w817) -> (ceil(x): smallest int >= x=w816:dbl)
              n1748 = local write "ImageSlide"(w816) -> ()
            }
          }
          n1749 = case shown="True" "Zero 2" {
            tunnel: [w812 w813] -> w512
            frame False {
              n1750 = global read "GlobelFSCOPE.vi" "Focus"() -> (w812:dbl)
            }
            frame True {
              w813 = 0.0 ("Focus")
              n1751 = global write "GlobelFSCOPE.vi" "Focus"(w813) -> ()
            }
          }
          "Focus" <- w512
          n1752 = property on="Image 1" class="IntGraph (strict)"("Y Scale.Range:Maximum"=w499) -> ()  [unwired: 2 in, 2 out]
          n1753 = property on="ImageSlide" class="Slide (strict)"("Scale.Range:Minimum"=0.0, "Scale.Range:Maximum"=w530, "Visible"=w534) -> ()  [unwired: 2 in, 2 out]
          n1754 = Wait (ms)(milliseconds to wait=u32 40) -> ()  [unwired: 1 out]
          "Ready?" <- TRUE ("Ready?")
        }
        "Intensity" <- w397
      }
    }
    n1755 = local read "ParametersFScope"() -> (w220:T7)
    n1756 = local read "scans to read"() -> (w221:sgl)
    n1757 = local read "ScaleCluster"() -> (w222:T3)
    n1758 = Bundle("ScaleCluster"=w222, "scans to read"=w221) -> (w219:T20)  [unwired: 1 in]
    n1759 = call "ScaleScanlineFScope.vi"("Parameters"=w220, "ScaleCluster"=w219) -> ("ScanlineScaled"=w214:dbl[][])
    n1760 = case shown="True" w209 {
      tunnel: [w339 w342] -> w210
      frame False {
        n1761 = local read "line scan time (ms)"() -> (w341:sgl)
        n1762 = local read "total y pixels"() -> (w340:sgl)
        n1763 = Multiply(x=w341, y=w340) -> (x*y=w339:sgl)
      }
      frame True {
        n1764 = local read "Pixel Clock (Hz) FScope"() -> (w344:sgl)
        n1765 = local read "scans to read"() -> (w343:sgl)
        n1766 = Divide(x=w343, y=w344) -> (x/y=w342:sgl)
      }
    }
    n1767 = local read "Number of frames"() -> (w212:sgl)
    n1768 = local read "Averaging"() -> (w213:u16)
    n1769 = Compound Arithmetic op=MULTIPLY(w212, w213, w210) -> (w211:sgl)
    n1770 = case shown="True" w295 {
      tunnel: w286 -> [w3059 w3266]
      tunnel: w285 -> [w3060 w3265]
      tunnel: w289 -> [w3058 w3242]
      tunnel: w259 -> [w3057 w3243]
      tunnel: w297 -> [w3054 w3293]
      tunnel: w261 -> [w3055 w3292]
      tunnel: w296 -> [w3056 w3291]
      tunnel: [w3054 w3290] -> w267
      tunnel: [w3055 w3289] -> w266
      tunnel: [w3056 w3288] -> w265
      tunnel: [w3057 w3287] -> w277
      tunnel: [w3058 w3286] -> w279
      tunnel: [w3059 w3285] -> w269
      tunnel: [w3060 w3268] -> w270
      tunnel: [w3052 w3248] -> w293
      tunnel: [w3053 w3249] -> w292
      tunnel: w291 -> [w3053 w3277]
      tunnel: w290 -> [w3052 w3279]
      tunnel: w260 -> [w3051 w3241]
      tunnel: w284 -> [w3050 w3240]
      tunnel: [w3051 w3271] -> w271
      tunnel: [w3050 w3270] -> w223
      tunnel: w276 -> [w3046 w3257]
      tunnel: w275 -> [w3045 w3256]
      tunnel: [w3046 w3255] -> w273
      tunnel: [w3045 w3254] -> w272
      tunnel: w263 -> [w3044 w3253]
      tunnel: [w3044 w3229] -> w198
      tunnel: w220 -> [_ w3237]
      tunnel: w214 -> [_ w3236]
      tunnel: w219 -> [_ w3235]
      tunnel: w218 -> [w3042 w3234]
      tunnel: w217 -> [w3043 w3233]
      tunnel: [w3042 w3232] -> w215
      tunnel: [w3043 w3231] -> w216
      tunnel: w211 -> [_ w3230]
      tunnel: w175 -> [w3039 w3228]
      tunnel: w185 -> [w3038 w3227]
      tunnel: [w3041 w3226] -> w190
      tunnel: [w3040 w3225] -> w189
      tunnel: [w3034 w3224] -> w188
      tunnel: [w3035 w3223] -> w187
      tunnel: w170 -> [w3037 w3222]
      tunnel: w186 -> [w3036 w3221]
      tunnel: w166 -> [_ w3199]
      tunnel: [w3033 w3199] -> w163
      tunnel: w162 -> [w3033 _]
      tunnel: w160 -> [w3032 _]
      frame False {
        n1771 = local write "Ready?"(FALSE ("Ready?")) -> ()
        n1772 = local write "Save?"(FALSE ("Save?")) -> ()
        n1773 = local read "Open?"() -> (w3049:bool)
        n1774 = case shown="False" w3049 {
          tunnel: [w3065 w3141] -> w3041
          tunnel: [w3067 w3140] -> w3040
          tunnel: w3039 -> [w3066 _]
          tunnel: w3038 -> [w3068 _]
          tunnel: [w3069 w3139] -> w3035
          tunnel: [w3070 w3138] -> w3034
          tunnel: w3037 -> [w3070 _]
          tunnel: w3036 -> [w3069 _]
          tunnel: w3032 -> [w3061 _]
          frame False {
            n1775 = local read "Channel selector"() -> (w3062:u8)
            n1776 = Greater Or Equal?(x=w3062, y=u16 3) -> (x >= y?=w3063:bool)
            n1777 = And(x=w3061, y=w3063) -> ()  [unwired: 1 out]
            n1778 = case shown="True" w3061 {
              tunnel: w3066 -> [w3071 _]
              tunnel: w3068 -> [w3072 _]
              tunnel: [w3072 w3077] -> w3067
              tunnel: [w3071 w3076] -> w3065
              tunnel: w3062 -> [_ w3078]
              frame False {
              }
              frame True {
                w3101 = 1  # bytes/DBL
                w3103 = u8 0  # type U8
                n1779 = property on="Property Node" class="VI"() -> ("VI Path"=w3090:path)  [unwired: 2 in, 2 out]
                n1780 = Strip Path(path=w3090) -> (stripped path=w3091:path)  [unwired: 1 out]
                n1781 = Build Path(base path=w3091, name or relative path="Stack.tmp") -> (appended path=w3088:path)
                n1782 = Open/Create/Replace File "Open File"(file path (use dialog)=w3088) -> (refnum out=w3073:refnum<file>, error out=w3074:errorcluster)  [unwired: 5 in, 1 out]
                n1783 = Deny Access(4:w3074, 6:T12."deny write-only" ("deny mode (2)"), 7:w3073) -> (0:w3097:errorcluster, 3:w3098:refnum<file>)
                n1784 = Get File Size "EOF"(file=w3098, error in=w3097) -> (refnum out=w3104:refnum<file>, size (in bytes)=w3075:i64, 0:w3099:errorcluster)
                n1785 = To Long Integer(number=w3075) -> (32bit integer=w3102:i32)
                n1786 = Quotient & Remainder(x=w3102, y=w3101) -> (floor(x/y)=w3100:i32)  [unwired: 1 out]
                n1787 = local read "X-pixels"() -> (w3082:sgl)
                n1788 = Read from Binary File "Read File"(5:w3103, 8:w3099, 10:w3100, 11:w3104) -> (0:w3092:errorcluster, 2:w3095:u8[], 3:w3093:refnum<file>)  [unwired: 2 in, 1 out]
                n1789 = Array Subset(array=w3095, index=768) -> (w3080:u8[])  [unwired: 1 in]
                n1790 = case shown="0, Default" w3078 {
                  tunnel: [w3108 w3111 w3112 w3115 w3119 w3123] -> w3081
                  tunnel: w3080 -> [w3107 w3110 w3114 w3117 w3120 w3122]
                  tunnel: [w3106 w3109 w3113 w3116 w3118 w3121] -> w3079
                  frame 1 {
                    n1791 = Decimate 1D Array(w3107) -> (w3108:u8[], w3106:u8[])
                  }
                  frame 2 {
                    n1792 = Decimate 1D Array(w3110) -> (w3111:u8[], w3109:u8[])
                  }
                  frame 3 {
                    n1793 = Decimate 1D Array(w3114) -> (w3113:u8[], w3112:u8[])  [unwired: 1 out]
                  }
                  frame 4 {
                    n1794 = Decimate 1D Array(w3117) -> (w3115:u8[], w3116:u8[])  [unwired: 1 out]
                  }
                  frame 5 {
                    n1795 = Decimate 1D Array(w3120) -> (w3118:u8[], w3119:u8[])  [unwired: 1 out]
                  }
                  frame 0, Default {
                    n1796 = Decimate 1D Array(w3122) -> (w3123:u8[], w3121:u8[])
                  }
                }
                n1797 = Array Size(array=w3081) -> (size(s)=w3083:i32)
                n1798 = Divide(x=w3083, y=w3082) -> (x/y=w3084:sgl)
                n1799 = Close File(refnum=w3093, error in=w3092) -> (error out=w3094:errorcluster)  [unwired: 1 out]
                n1800 = Round To Nearest(number=w3084) -> (nearest integer value=w3087:sgl)
                n1801 = call <vilib>:"Simple Error Handler.vi"("error in (no error)"=w3094) -> ()  [unwired: 4 in, 5 out]
                n1802 = Reshape Array(w3081, w3087, w3082) -> (w3085:u8[][])
                n1803 = Reshape Array(w3079, w3087, w3082) -> (w3086:u8[][])
                n1804 = Transpose 2D Array(2D array=w3085) -> (transposed array=w3076:u8[][])
                n1805 = Transpose 2D Array(2D array=w3086) -> (transposed array=w3077:u8[][])
              }
            }
          }
          frame True {
            w3173 = u16 1 items=["focus", "frame", "line", "user-defined line", "3D user-defined line"] ("frame/line indicator")
            w3188 = u16 0 items=["user-defined frame", "64 x 64, 2ms lines", "128 x 128, 2ms lines", "256 x 256, 2ms lines", "512 x 512, 2ms lines", "32 x 32, 1ms lines"] ("Scan format")
            n1806 = call "LoadImagesnewFOCUS.vi"() -> ("Image2Array"=w3140:u8[][], "Image1Array"=w3141:u8[][], "HeaderCluster"=w3198:T21, "Zsin3D"=w3187:sgl[], "ScanLine FreeLine"=w3146:sgl[][], "Image4Array"=w3139:u8[][], "Image3Array"=w3138:u8[][])
            n1807 = Transpose 2D Array(2D array=w3146) -> (transposed array=w3145:sgl[][])
            n1808 = local write "Zsin3D"(w3187) -> ()
            n1809 = local write "ScanLineFreeLine"(w3145) -> ()
            n1810 = local write "frame/line indicator"(w3173) -> ()
            n1811 = local write "Scan format"(w3188) -> ()
            n1812 = Unbundle(w3198) -> ("Program Version"=w3159:u16, "name"=w3197:string, "Time"=w3196:string, "Date"=w3195:string, "start"=w3194:u32, "stop"=w3193:u32, "IntDevUsed"=w3192:bool, "Intensity"=w3191:sgl, "Scan Block Length"=w3190:sgl, "Pixel Clock (Hz)"=w3189:sgl, "X-pixels"=w3157:sgl, "Y-lines"=w3156:sgl, "Number of frames"=w3137:sgl, "Averaging"=w3136:u16, "line scan time (ms)"=w3135:sgl, "Retrace pixels"=w3134:sgl, "z-step (um)"=w3133:sgl, "x-step (um)"=w3132:sgl, "y-step (um)"=w3131:sgl, "x jog"=w3130:sgl, "y jog"=w3129:sgl, "Rotation"=w3128:sgl, "Zoom"=w3127:sgl, "Number of stacks"=w3126:sgl, "Time interval [s]"=w3125:sgl, w3124:T22)  [unwired: 2 out]
            n1813 = Type Cast(type="" ("concatenated string"), x=w3159) -> (*(type *) &x=w3164:string)
            n1814 = local write "Number of Stacks"(w3126) -> ()
            n1815 = local write "Time interval [s]"(w3125) -> ()
            n1816 = String Subset(string=w3164, offset (0)=0, length (rest)=1 ("length (rest)")) -> (substring=w3163:string)
            n1817 = String Subset(string=w3164, offset (0)=1, length (rest)=1 ("length (rest)")) -> (substring=w3162:string)
            n1818 = Concatenate Strings(w3163, "." ("concatenated string"), w3162) -> (w3160:string)
            n1819 = local write "Number of stacks"(w3126) -> ()
            n1820 = local write "Time interval [s]"(w3125) -> ()
            n1821 = local write "Program Version"(w3160) -> ()
            n1822 = local write "Filename"(w3197) -> ()
            n1823 = local write "Number of frames"(w3137) -> ()
            n1824 = local write "Averaging"(w3136) -> ()
            n1825 = local write "Program Version"(w3159) -> ()
            n1826 = local write "Time"(w3196) -> ()
            n1827 = local write "Date"(w3195) -> ()
            n1828 = local write "start"(w3194) -> ()
            n1829 = local write "stop"(w3193) -> ()
            n1830 = local write "IntDevUsed"(w3192) -> ()
            n1831 = local write "Intensity"(w3191) -> ()
            n1832 = local write "Scan Block Length"(w3190) -> ()
            n1833 = local write "Pixel Clock (Hz)"(w3189) -> ()
            n1834 = local write "X-pixels"(w3157) -> ()
            n1835 = local write "Y-lines"(w3156) -> ()
            n1836 = local write "line scan time (ms)"(w3135) -> ()
            n1837 = local write "x-step (um)"(w3132) -> ()
            n1838 = local write "y-step (um)"(w3131) -> ()
            n1839 = local write "x jog"(w3130) -> ()
            n1840 = local write "y jog"(w3129) -> ()
            n1841 = local write "Rotation"(w3128) -> ()
            n1842 = local write "Zoom"(w3127) -> ()
            n1843 = local write "Retrace pixels"(w3134) -> ()
            n1844 = local write "z-step (um)"(w3133) -> ()
            n1845 = local write "Y dim"(w3156) -> ()
            n1846 = local write "X dim"(w3157) -> ()
            n1847 = local write "Averaging"(w3136) -> ()
            n1848 = local write "Number of Frames"(w3137) -> ()
